vi "DtOLReadMultiple2DU32.vi"(5 "Number Chan to Read":u32, 6 "Buffer size":i32, 7 "OnlyReadAvailable":bool, 8 "error in (no error)":errorcluster, 9 "Timeout":dbl=10.0, 10 "Samples Per Channel":i32=-1, 11 "Task in":i32) -> (0 "error out":errorcluster, 1 "Num Samples Per Channel Read":u32, 2 "2D Data out":u32[][](array[numeric]), 3 "Task out":i32, 4 "Num Channels Read":u32)   [LabVIEW 2016]
doc: "Reads multiple samples from multiple virtual channels of a task you specify, and returns the data as a two-dimensional array of unsigned, 32-bit numbers. This VI is typically used with analog input tasks that use the DtOLTiming (Input - Set Timing) VI."
uses:
  <userlib>/LV-Link3/DtLvLink.lvlib
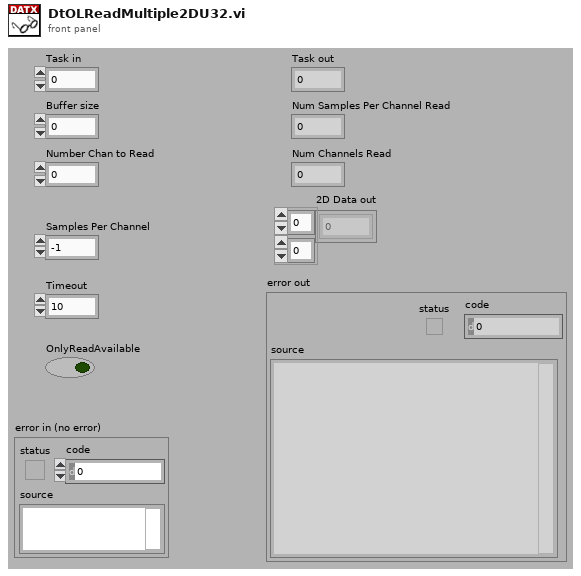
[diagram p1: front panel]
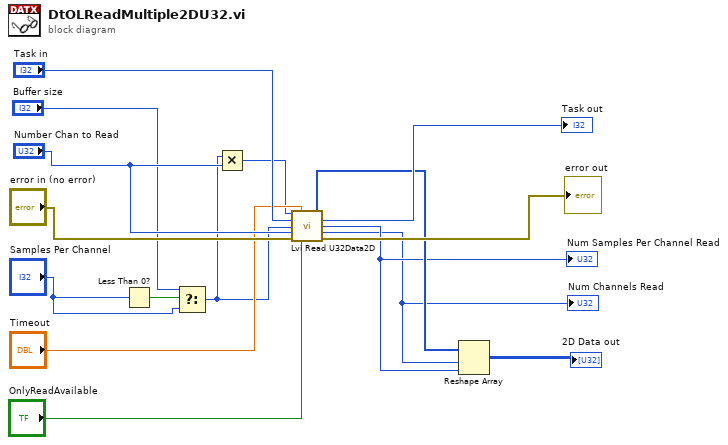
[diagram p0: block diagram]
diagram:
  n1 = Less Than 0?(x="Samples Per Channel") -> (x < 0?=w9:bool)
  n2 = Select(t="Buffer size", s=w9, f="Samples Per Channel") -> (s? t:f=w6:i32)
  n3 = Multiply(x=w6, y="Number Chan to Read") -> (x*y=w5:u32)
  n4 = call <userlib>:"Lvi Read U32Data2D.vi"("DataBufSize"=w5, "timeout"="Timeout", "TaskRef"="Task in", "PointsPerChan"=w6, "NumChansToRead"="Number Chan to Read", "error in (no error)"="error in (no error)", "OnlyReadAvailable"="OnlyReadAvailable") -> ("DataBuf"=w4:u32[], "TaskRef out"=→"Task out":i32, "PointsPerChan out"=w2:u32, "NumChansToRead out"=w1:u32, "error out"=→"error out":errorcluster)  [unwired: 2 in, 2 out]
  "Num Samples Per Channel Read" <- w2
  "Num Channels Read" <- w1
  n5 = Reshape Array "Reshape Array"(w4, w1, w2) -> (→"2D Data out":u32[][])
